vi "OAT Order Power Spectrum.vi"   [LabVIEW 2017, in "SoundVib_OrderTracking.lvlib"]
doc: "Computes the order power spectrum of an even-angle signal. Wire data to the <B>even-angle signal</B> input to determine the polymorphic instance to use or manually select the instance."
uses:
  <vilib>/addons/Sound and Vibration/Order Analysis/Resample Order Tracking/SoundVib_OrderTracking.lvlib
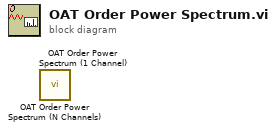
[diagram p0: block diagram]
diagram:
  n1 = call <vilib>:"OAT Order Power Spectrum (N Channels).vi"() -> ()  [unwired: 9 in, 7 out]
  n2 = call <vilib>:"OAT Order Power Spectrum (1 Channel).vi"() -> ()  [unwired: 9 in, 7 out]
